vi "二进制解析-8.6.vi"(3 "索引":i32=5, 4 "数值":i32 format="%x") -> (0 "连接的字符串":string, 1 "低位子数组":i32[](array[numeric]), 2 "高位子数组":i32[](array[numeric]))   [LabVIEW 2013]
panel:
  out "数组":i32[](array[numeric])
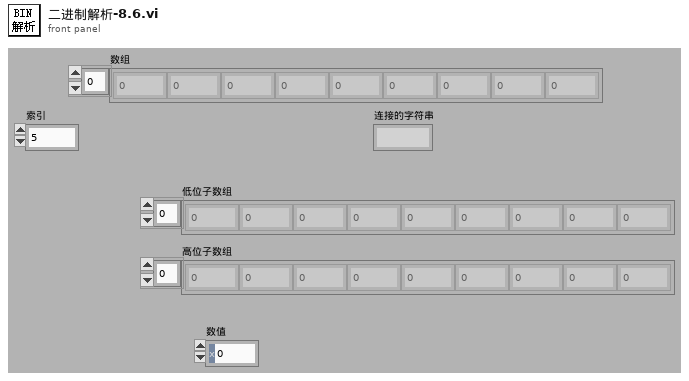
[diagram p1: front panel]
types:
  T1 = cluster{"[0]":i32, "[1]":i32, "[2]":i32, "[3]":i32, "[4]":i32, "[5]":i32, "[6]":i32, "[7]":i32, "[8]":i32}
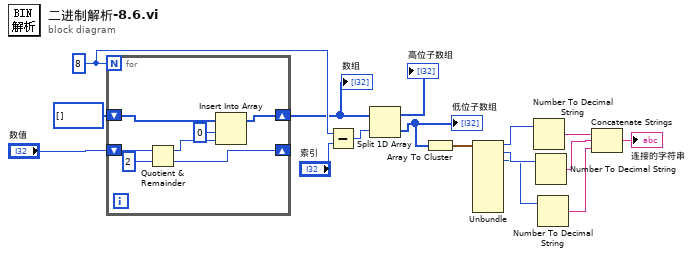
[diagram p0: block diagram]
diagram:
  w4 = 8
  n1 = for {
    N: w4 -> [_]
    shift-right: [w20] -> w2
    shift-left: i32[] [] -> [w21]
    shift-right: [w17] -> _
    shift-left: "数值" -> [w23]
    n2 = Quotient & Remainder(x=w23, y=2) -> (x-y*floor(x/y)=w18:i32, floor(x/y)=w17:i32)
    n3 = Insert Into Array(array=w21, index=0 ("索引"), new element=w18) -> (w20:i32[])
  }
  "数组" <- w2
  n4 = Subtract(x=w4, y="索引") -> (x-y=w3:i32)
  n5 = Split 1D Array(array=w2, index=w3) -> (first subarray=→"高位子数组":i32[], second subarray=w14:i32[])
  "低位子数组" <- w14
  n6 = Array To Cluster(array=w14) -> (cluster=w13:T1)
  n7 = Unbundle(w13) -> ("[0]"=w12:i32, "[1]"=w11:i32, "[2]"=w10:i32)  [unwired: 6 out]
  n8 = Number To Decimal String(number=w12) -> (decimal integer string=w9:string)  [unwired: 1 out]
  n9 = Number To Decimal String(number=w11) -> (decimal integer string=w8:string)  [unwired: 1 out]
  n10 = Number To Decimal String(number=w10) -> (decimal integer string=w7:string)  [unwired: 1 out]
  n11 = Concatenate Strings(w9, w8, w7) -> (→"连接的字符串":string)
